vi "Esame sub.vi"() -> (0 "N":i32)   [LabVIEW 2012]
panel:
  out "5 cifre significative (negativo)":string
  out "Numero di presenze":i32
  out "5 cifre significative":string
  out "Numero":dbl
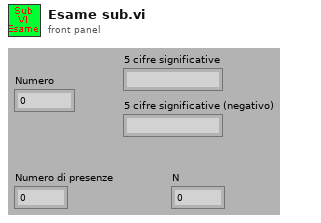
[diagram p1: front panel]
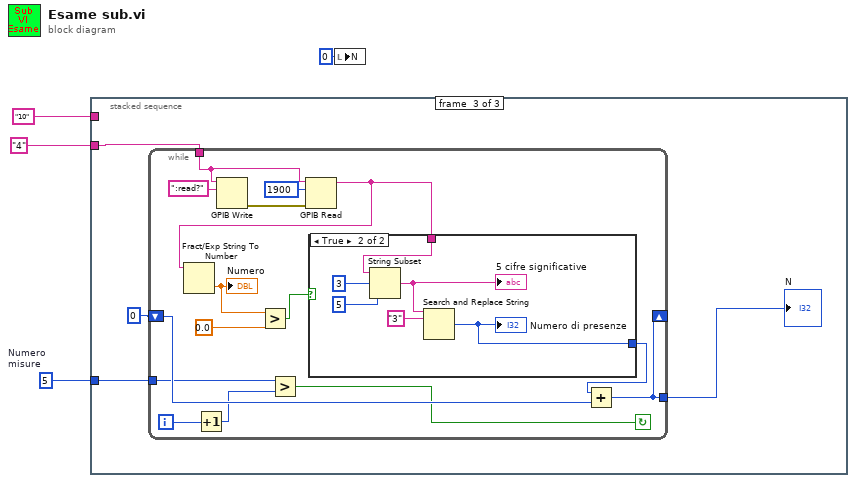
[diagram p0: block diagram]
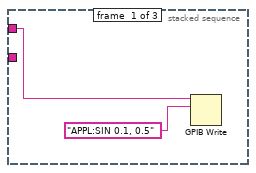
[diagram p2: hidden frame]
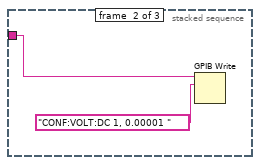
[diagram p3: hidden frame]
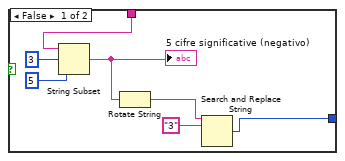
[diagram p4: hidden frame]
diagram:
  w2 = 5  # Numero misure
  n1 = stacked-sequence {
    tunnel: "10" -> [w6 _ _]
    tunnel: "4" -> [_ w8 w10]
    tunnel: w2 -> [_ _ w12]
    frame #0 {
      n2 = GPIB Write(0:w6, 1:"APPL:SIN 0.1, 0.5" ("data")) -> ()  [unwired: 3 in, 2 out]
    }
    frame #1 {
      n3 = GPIB Write(0:w8, 1:"CONF:VOLT:DC 1, 0.00001 " ("data")) -> ()  [unwired: 3 in, 2 out]
    }
    frame #2 {
      n4 = while {
        tunnel: w12 -> [w16]
        shift-right: [w14] -> _
        shift-left: 0 -> [w19]
        tunnel: w10 -> [w13]
        tunnel: [w14] -> w9
        i -> [w18]
        stop <- w15 continue-if-true
        n5 = Increment(x=w18) -> (x+1=w17:i32)
        n6 = GPIB Write(0:w13, 1:":read?" ("data")) -> (6:w27:errorcluster)  [unwired: 3 in, 1 out]
        n7 = Greater?(x=w16, y=w17) -> (0:w15:bool)
        n8 = GPIB Read(0:w13, 1:1900 ("byte count"), 3:w27) -> (5:w21:string)  [unwired: 2 in, 2 out]
        n9 = Fract/Exp String To Number(string=w21) -> (number=w24:dbl)  [unwired: 3 in, 1 out]
        "Numero" <- w24
        n10 = Greater?(x=w24, y=0.0) -> (0:w22:bool)
        n11 = case shown="True" w22 {
          tunnel: w21 -> [w34 w38]
          tunnel: [w28 w35] -> w20
          frame False {
            n12 = String Subset(string=w34, offset (0)=3, length (rest)=5 ("length (rest)")) -> (substring=w31:string)
            "5 cifre significative (negativo)" <- w31
            n13 = Rotate String(1:w31) -> (0:w29:string)
            n14 = Search and Replace String(input string=w29, search string="3") -> (number of replacements=w28:i32)  [unwired: 6 in, 3 out]
          }
          frame True {
            n15 = String Subset(string=w38, offset (0)=3, length (rest)=5 ("length (rest)")) -> (substring=w37:string)
            "5 cifre significative" <- w37
            n16 = Search and Replace String(input string=w37, search string="3") -> (number of replacements=w35:i32)  [unwired: 6 in, 3 out]
            "Numero di presenze" <- w35
          }
        }
        n17 = Add(x=w20, y=w19) -> (x+y=w14:i32)
      }
      "N" <- w9
    }
  }
  n18 = local write "N"(0 ("N")) -> ()
